vi "record_tsv_CCP.vi"(0 "use_nfs_disk_also":bool=TRUE, 2 "use_date_folder":bool=TRUE, 3 "logging_on":bool=TRUE, 5 "file_name":string="record", 6 "error in":errorcluster, 7 "folder_name":string="subsystem", 8 "format_array":string[](array[string]), 9 "value_array":dbl[](array[numeric])=[0.0], 11 "time":timestamp) -> (4 "error out":errorcluster)   [LabVIEW 2019]
uses:
  <vilib>/Utility/file.llb/Write Delimited Spreadsheet (string).vi
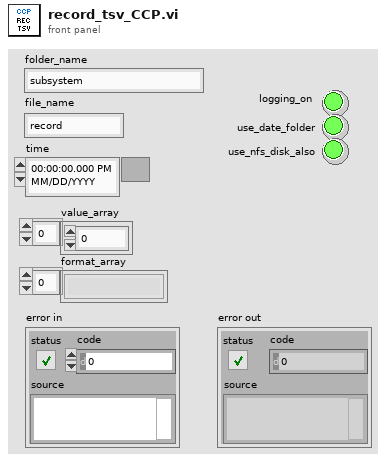
[diagram p1: front panel]
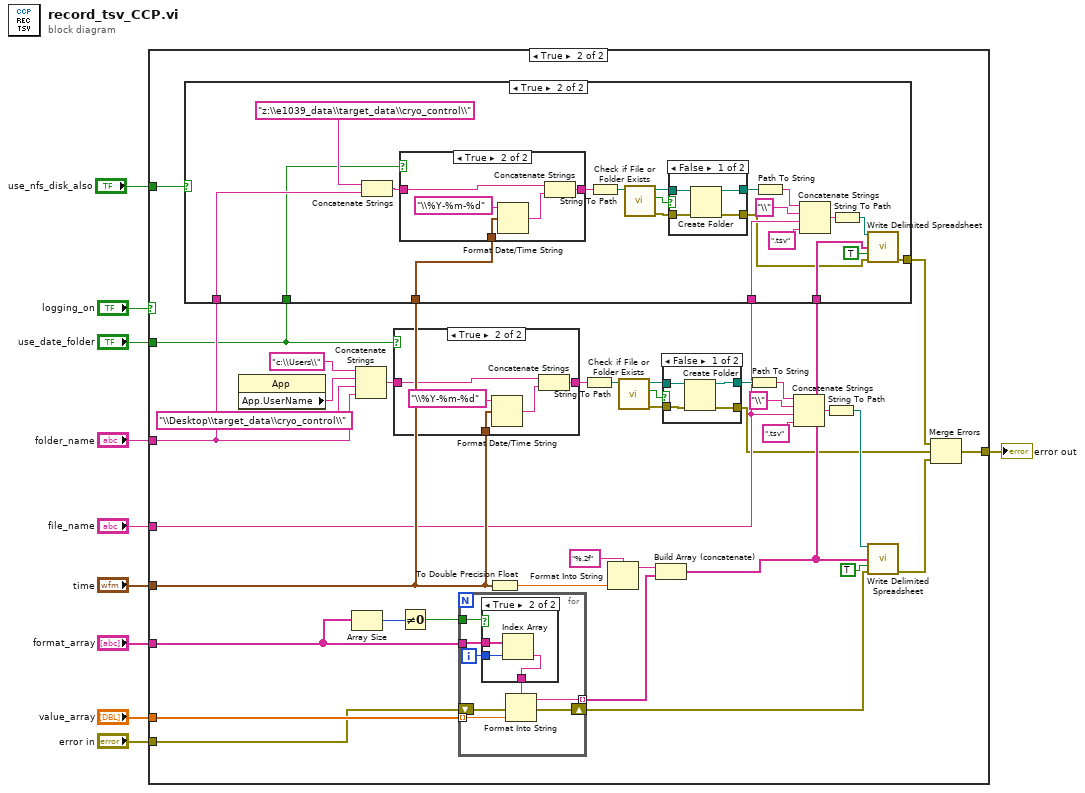
[diagram p0: block diagram]
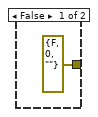
[diagram p3: hidden frame]
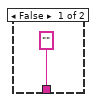
[diagram p7: hidden frame]
diagram:
  n1 = case shown="True" "logging_on" {
    tunnel: "file_name" -> [_ w20]
    tunnel: "folder_name" -> [_ w22]
    tunnel: "value_array" -> [_ w31]
    tunnel: [w11 w16] -> w7
    tunnel: "format_array" -> [_ w27]
    tunnel: "use_date_folder" -> [_ w18]
    tunnel: "time" -> [_ w21]
    tunnel: "error in" -> [w11 w24]
    tunnel: "use_nfs_disk_also" -> [_ w17]
    frame False {
    }
    frame True {
      n2 = property class="App"() -> ("App.UserName"=w44:string)  [unwired: 2 in, 2 out]
      n3 = Array Size(array=w27) -> (size(s)=w26:i32)
      n4 = Concatenate Strings("c:\\Users\\", w44, "\\Desktop\\target_data\\cryo_control\\", w22) -> (w29:string)
      n5 = case shown="True" w18 {
        tunnel: w29 -> [w82 w87]
        tunnel: [w82 w86] -> w28
        tunnel: w21 -> [_ w85]
        frame False {
        }
        frame True {
          n6 = Format Date/Time String(time format string (%c)="\\%Y-%m-%d", seconds (now)=w85) -> (date/time string=w83:string)  [unwired: 1 in]
          n7 = Concatenate Strings(w87, w83) -> (w86:string)
        }
      }
      n8 = Not Equal To 0?(x=w26) -> (x != 0?=w25:bool)
      n9 = for {
        tunnel: [w95] -> w30 mode=indexing
        tunnel: w31 -> [w94] mode=indexing
        tunnel: w27 -> [w91]
        tunnel: w25 -> [w93]
        shift-right: [w89] -> w23
        shift-left: w24 -> [w90]
        i -> [w88]
        n10 = case shown="True" w93 {
          tunnel: ["" w99] -> w92
          tunnel: w91 -> [_ w98]
          tunnel: w88 -> [_ w97]
          frame False {
          }
          frame True {
            n11 = Index Array(array=w98, index=w97) -> (element=w99:string)
          }
        }
        n12 = Format Into String(format string=w92, error in=w90, w94) -> (resulting string=w95:string, error out=w89:errorcluster)  [unwired: 1 in]
      }
      n13 = To Double Precision Float(number=w21) -> (double precision float=w33:dbl)
      n14 = String To Path(string=w28) -> (path=w39:path)
      n15 = Format Into String(format string="%.2f", w33) -> (resulting string=w47:string)  [unwired: 2 in, 1 out]
      n16 = call <vilib>:"Check if File or Folder Exists.vi"("path"=w39) -> ("error out"=w15:errorcluster, "file or folder exists?"=w38:bool, "dup path"=w36:path)  [unwired: 8 in]
      n17 = Build Array (concatenate)(w47, w30) -> (w19:string[])
      n18 = case shown="True" w17 {
        tunnel: w22 -> [_ w58]
        tunnel: w21 -> [_ w57]
        tunnel: w20 -> [_ w56]
        tunnel: w19 -> [_ w53]
        tunnel: w18 -> [_ w52]
        tunnel: [errorcluster {"status"=FALSE, "code"=0, "source"=""} ("error out") w49] -> w12
        frame False {
        }
        frame True {
          n19 = Concatenate Strings("z:\\e1039_data\\target_data\\cryo_control\\", w58) -> (w60:string)
          n20 = case shown="True" w52 {
            tunnel: w60 -> [w70 w75]
            tunnel: [w70 w74] -> w59
            tunnel: w57 -> [_ w73]
            frame False {
            }
            frame True {
              n21 = Format Date/Time String(time format string (%c)="\\%Y-%m-%d", seconds (now)=w73) -> (date/time string=w71:string)  [unwired: 1 in]
              n22 = Concatenate Strings(w75, w71) -> (w74:string)
            }
          }
          n23 = String To Path(string=w59) -> (path=w65:path)
          n24 = call <vilib>:"Check if File or Folder Exists.vi"("path"=w65) -> ("error out"=w51:errorcluster, "file or folder exists?"=w64:bool, "dup path"=w62:path)  [unwired: 8 in]
          n25 = case shown="False" w64 {
            tunnel: w62 -> [w79 w81]
            tunnel: [w78 w81] -> w63
            tunnel: w51 -> [w77 w80]
            tunnel: [w76 w80] -> w50
            frame False {
              n26 = Create Folder(path (use dialog)=w79, error in=w77) -> (created path=w78:path, error out=w76:errorcluster)  [unwired: 1 in, 1 out]
            }
            frame True {
            }
          }
          n27 = Path To String(path=w63) -> (string=w61:string)
          n28 = Concatenate Strings(w61, "\\", w56, ".tsv" ("string")) -> (w66:string)
          n29 = String To Path(string=w66) -> (path=w55:path)
          n30 = call-poly <vilib>:"Write Delimited Spreadsheet.vi"("file path (dialog if empty)"=w55, "1D data"=w53, "append to file? (new file:F)"=TRUE, "error in (no error)"=w50) -> ("error out"=w49:errorcluster)  [unwired: 10 in, 1 out]
        }
      }
      n31 = case shown="False" w38 {
        tunnel: w36 -> [w103 w105]
        tunnel: [w102 w105] -> w37
        tunnel: w15 -> [w101 w104]
        tunnel: [w100 w104] -> w14
        frame False {
          n32 = Create Folder(path (use dialog)=w103, error in=w101) -> (created path=w102:path, error out=w100:errorcluster)  [unwired: 1 in, 1 out]
        }
        frame True {
        }
      }
      n33 = Path To String(path=w37) -> (string=w35:string)
      n34 = Concatenate Strings(w35, "\\", w20, ".tsv" ("string")) -> (w40:string)
      n35 = String To Path(string=w40) -> (path=w34:path)
      n36 = call-poly <vilib>:"Write Delimited Spreadsheet.vi"("file path (dialog if empty)"=w34, "1D data"=w19, "append to file? (new file:F)"=TRUE, "error in (no error)"=w23) -> ("error out"=w13:errorcluster)  [unwired: 10 in, 1 out]
      n37 = Merge Errors(w12, w14, w13) -> (w16:errorcluster)
    }
  }
  "error out" <- w7
